vi "Initialise - From Table.vi"(4 "Keep Original Tag":bool, 6 "Tag Root":string, 8 "error in (no error)":errorcluster, 9 "Aliased Tags":T1[](array[typedef]), 10 "Buses":refnum<class "Bus_Access.lvclass">[](array[class]), 11 "Remap Bus in":refnum<class "Alias Bus.lvclass">) -> (0 "error out":errorcluster, 3 "Remap Bus out":refnum<class "Alias Bus.lvclass">)   [LabVIEW 2021, in "Alias Bus.lvclass"]
uses:
  Alias Bus.lvclass
  C:/TSA/Omni-Bus/Source/Omni-Bus/Bus Access/Bus_Access.lvclass
  Omni-Bus/Bus Access/Bus_Access.lvclass
  Support/Remap Table Type.ctl
  Support/Remap Type.ctl
  Alias Bus.lvclass/Alias Bus.ctl
  Omni-Bus/Bus Access/Bus_Access.lvclass/Bus_Access.ctl
  Properties/Write Buses.vi
  Properties/Write Map.vi
  Omni-Bus/Bus Access/Properties/Write Tag Root.vi
  Properties/Write Keep Original.vi
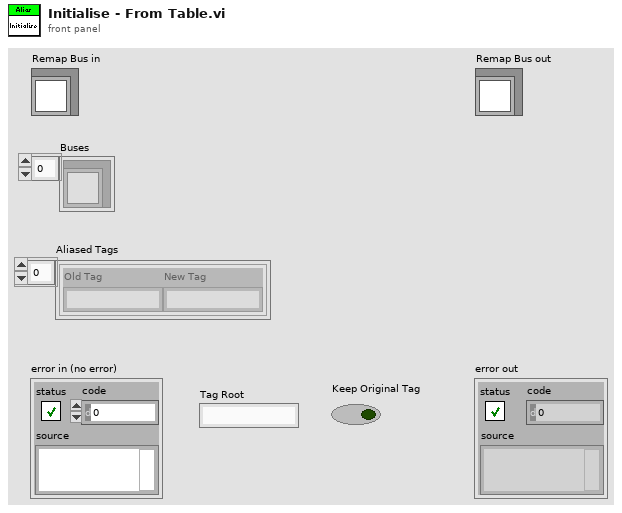
[diagram p1: front panel]
types:
  T1 = typedef "Alias Bus.lvclass/Remap Table Type.ctl" = cluster{"Old Tag":string, "New Tag":string}
  T2 = typedef "Alias Bus.lvclass/Remap Type.ctl" = map{string, string}
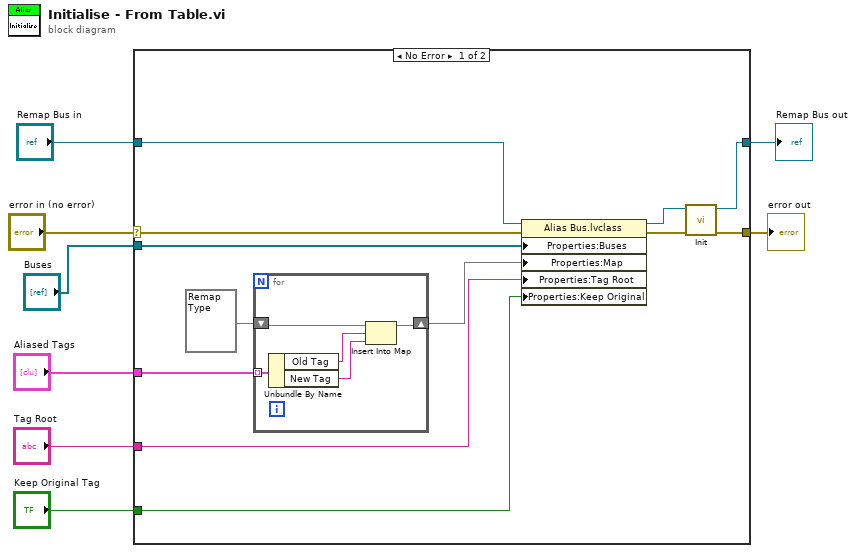
[diagram p0: block diagram]
diagram:
  n1 = case shown="No Error" "error in (no error)" {
    selector: "error in (no error)" -> [w20 w27]
    tunnel: [w11 w27] -> w7
    tunnel: [w9 w26] -> w5
    tunnel: "Remap Bus in" -> [w19 w26]
    tunnel: "Buses" -> [w18 _]
    tunnel: "Aliased Tags" -> [w17 _]
    tunnel: "Tag Root" -> [w14 _]
    tunnel: "Keep Original Tag" -> [w13 _]
    frame No Error {
      n2 = for {
        tunnel: w17 -> [w23] mode=indexing
        shift-right: [w24] -> w15
        shift-left: T2 {} ("Map") -> [w25]
        n3 = Unbundle By Name(w23) -> ("Old Tag"=w22:string, "New Tag"=w21:string)
        n4 = Insert Into Map(map in=w25, key=w22, value=w21) -> (map out=w24:T2)  [unwired: 2 out]
      }
      n5 = property class="Alias Bus.lvclass"(reference=w19, error in=w20, "Properties:Buses"=w18, "Properties:Map"=w15, "Properties:Tag Root"=w14, "Properties:Keep Original"=w13) -> (reference out=w10:refnum<class "Alias Bus.lvclass">, error out=w12:errorcluster)
      n6 = call-dynamic "Init.vi"("error in (no error)"=w12, "Data in"=w10) -> ("error out"=w11:errorcluster, "Data out"=w9:refnum<class "Alias Bus.lvclass">)  [unwired: 8 in]
    }
    frame Error {
    }
  }
  "error out" <- w7
  "Remap Bus out" <- w5
